vi "TrajectoryExecuteRelative.vi"(8 "Init":bool, 10 "End Relative\nOrientation Deg":dbl, 11 "Trajectory":T1 {"States"."POSE"."ROTATION"."SIN" format="%13.4f"; "States"."POSE"."ROTATION"."COS" format="%13.4f"; "States"."POSE"."ROTATION"."VALUE" format="%13.4f"; "States"."POSE"."TRANSLATION"."Y" format="%14.3f"; "States"."POSE"."TRANSLATION"."X" format="%14.3f"; "TotalTImeSecs" format="%20.3f"}) -> (0 "AtReference":bool, 2 "Done":bool, 3 "Chassis Velocity Target Met,Met,Rad":T6 {"vOmega" format="%10.3f"; "vY" format="%10.3f"; "vX" format="%10.3f"})   [LabVIEW 2023]
uses:
  <vilib>/Rock Robotics/WPI/ThirdParty/JAS_Junk/TrajLib/TypeDef/CHASSIS_SPEEDS.ctl
  <vilib>/Rock Robotics/WPI/ThirdParty/JAS_Junk/TrajLib/TypeDef/TRAJECTORY.ctl
  <vilib>/Rock Robotics/WPI/ThirdParty/JAS_Junk/TrajLib/TypeDef/TRAJ_STATE.ctl
  <vilib>/Rock Robotics/WPI/ThirdParty/JAS_Junk/TrajLib/TypeDef/POSE2D.ctl
  <vilib>/Rock Robotics/WPI/ThirdParty/JAS_Junk/TrajLib/TypeDef/TRANSLATION2D.ctl
  <vilib>/Rock Robotics/WPI/ThirdParty/JAS_Junk/TrajLib/TypeDef/ROTATION2D.ctl
  <vilib>/Rock Robotics/WPI/ThirdParty/JAS_Junk/TrajLib/VI/Util_GetTime_U32.vi
  <vilib>/Rock Robotics/WPI/ThirdParty/JAS_Junk/TrajLib/SwerveOdometry_UpdateX.vi
  <vilib>/Rock Robotics/WPI/ThirdParty/JAS_Junk/TrajLib/SwerveOdometry_ResetPosition.vi
  <vilib>/Rock Robotics/WPI/ThirdParty/JAS_Junk/TrajLib/SwerveOdometry_New.vi
  <vilib>/Rock Robotics/WPI/ThirdParty/JAS_Junk/TrajLib/HolDrvCtrl_New.vi
  <vilib>/Rock Robotics/WPI/ThirdParty/JAS_Junk/TrajLib/HolDrvCtrl_PackPID.vi
  <vilib>/Rock Robotics/WPI/ThirdParty/JAS_Junk/TrajLib/HolDrvCtrl_SetTolerance.vi
  <vilib>/Rock Robotics/WPI/ThirdParty/JAS_Junk/TrajLib/HolDrvCtrl_SetEnabled.vi
  <vilib>/Rock Robotics/WPI/ThirdParty/JAS_Junk/TrajLib/HolDrvCtrl_Calculate_Trajectory.vi
  <vilib>/Rock Robotics/WPI/ThirdParty/JAS_Junk/TrajLib/HolDrvCtrl_AtReference.vi
  <vilib>/Rock Robotics/WPI/ThirdParty/JAS_Junk/TrajLib/ProfiledPIDController_NewPeriod.vi
  <vilib>/Rock Robotics/WPI/ThirdParty/JAS_Junk/TrajLib/ProfiledPIDController_SetIntegratorRange.vi
  <vilib>/Rock Robotics/WPI/ThirdParty/JAS_Junk/TrajLib/ProfiledPIDController_DisableContInput.vi
  <vilib>/Rock Robotics/WPI/ThirdParty/JAS_Junk/TrajLib/ProfiledPIDController_EnableContInput.vi
  <vilib>/Rock Robotics/WPI/ThirdParty/JAS_Junk/TrajLib/TrapProfConstraint_New.vi
  <vilib>/Rock Robotics/WPI/ThirdParty/JAS_Junk/TrajLib/Translation2d_Create.vi
  <vilib>/Rock Robotics/WPI/ThirdParty/JAS_Junk/TrajLib/Rotation2d_Plus.vi
  <vilib>/Rock Robotics/WPI/ThirdParty/JAS_Junk/TrajLib/Twist2d_Create.vi
  <vilib>/Rock Robotics/WPI/ThirdParty/JAS_Junk/TrajLib/Rotation2d_Minus.vi
  <vilib>/Rock Robotics/WPI/ThirdParty/JAS_Junk/TrajLib/Pose2d_getTranslation.vi
  <vilib>/Rock Robotics/WPI/ThirdParty/JAS_Junk/TrajLib/Pose2d_New_TRRO.vi
  <vilib>/Rock Robotics/WPI/ThirdParty/JAS_Junk/TrajLib/VI/SwerveModulePosition_Get.vi
  <vilib>/Rock Robotics/WPI/ThirdParty/JAS_Junk/TrajLib/VI/SwerveModulePosition_New.vi
  <vilib>/Rock Robotics/WPI/ThirdParty/JAS_Junk/TrajLib/Twist2d_GetAll.vi
  <vilib>/Rock Robotics/WPI/ThirdParty/JAS_Junk/TrajLib/Pose2d_getRotation.vi
  <vilib>/Rock Robotics/SystemInterfaces/NetworkCommunication/NetComm_UsageReport_report.vi
  <vilib>/Rock Robotics/WPI/ThirdParty/JAS_Junk/TrajLib/PIDController_NewPeriod.vi
  <vilib>/Rock Robotics/WPI/ThirdParty/JAS_Junk/TrajLib/PIDController_SetIntegratorRange.vi
  <vilib>/Rock Robotics/WPI/ThirdParty/JAS_Junk/TrajLib/PIDController_Reset.vi
  <vilib>/Rock Robotics/WPI/ThirdParty/JAS_Junk/TrajLib/HolDrvCtrl_Calculate.vi
  <vilib>/Rock Robotics/WPI/ThirdParty/JAS_Junk/TrajLib/Pose2d_getXYAngle.vi
  <vilib>/Rock Robotics/WPI/ThirdParty/JAS_Junk/TrajLib/Rotation2d_GetRadians.vi
  <vilib>/Rock Robotics/WPI/ThirdParty/JAS_Junk/TrajLib/TrapProfState_New.vi
  <vilib>/Rock Robotics/WPI/ThirdParty/JAS_Junk/TrajLib/PIDController_DisableContinousInput.vi
  <vilib>/Rock Robotics/WPI/ThirdParty/JAS_Junk/TrajLib/PIDController_EnableContinousInput.vi
  <vilib>/Rock Robotics/WPI/ThirdParty/JAS_Junk/TrajLib/Rotation2d_RotateBy.vi
  <vilib>/Rock Robotics/WPI/ThirdParty/JAS_Junk/TrajLib/Rotation2d_UnaryMinus.vi
  <vilib>/Rock Robotics/WPI/ThirdParty/JAS_Junk/TrajLib/Rotation2d_GetAngleCosSin.vi
  <vilib>/Rock Robotics/WPI/ThirdParty/JAS_Junk/TrajLib/Pose2d_RelativeTo.vi
  <vilib>/Rock Robotics/WPI/ThirdParty/JAS_Junk/TrajLib/ProfiledPIDController_Calculate_Meas_Goal.vi
  <vilib>/Rock Robotics/WPI/ThirdParty/JAS_Junk/TrajLib/PIDController_Calculate_SP_PV.vi
  <vilib>/Rock Robotics/WPI/ThirdParty/JAS_Junk/TrajLib/ProfiledPIDController_Reset_PosOnly.vi
  <vilib>/Rock Robotics/WPI/ThirdParty/JAS_Junk/TrajLib/ChassisSpeeds_FromFieldRelativeSpeeds.vi
  <vilib>/Rock Robotics/WPI/ThirdParty/JAS_Junk/TrajLib/Rotation2d_CreateXY.vi
  <vilib>/Rock Robotics/WPI/ThirdParty/JAS_Junk/TrajLib/Transform2d_Create_PosePose.vi
  <vilib>/Rock Robotics/WPI/ThirdParty/JAS_Junk/TrajLib/ProfiledPIDController_SetGoal_PosOnly.vi
  <vilib>/Rock Robotics/WPI/ThirdParty/JAS_Junk/TrajLib/ProfiledPIDController_Calculate_Meas.vi
  <vilib>/Rock Robotics/WPI/ThirdParty/JAS_Junk/TrajLib/PIDController_SetSetpoint.vi
  <vilib>/Rock Robotics/WPI/ThirdParty/JAS_Junk/TrajLib/PIDController_Calculate_PV.vi
  <vilib>/Rock Robotics/WPI/ThirdParty/JAS_Junk/TrajLib/ProfiledPIDController_Reset.vi
  <vilib>/Rock Robotics/WPI/ThirdParty/JAS_Junk/TrajLib/Rotation2d_GetCos.vi
  <vilib>/Rock Robotics/WPI/ThirdParty/JAS_Junk/TrajLib/Rotation2d_GetSin.vi
  <vilib>/Rock Robotics/WPI/ThirdParty/JAS_Junk/TrajLib/Util_CalcDist.vi
  <vilib>/Rock Robotics/WPI/ThirdParty/JAS_Junk/TrajLib/Translation2d_RotateBy.vi
  <vilib>/Rock Robotics/WPI/ThirdParty/JAS_Junk/TrajLib/Translation2d_Minus.vi
  <vilib>/Rock Robotics/WPI/ThirdParty/JAS_Junk/TrajLib/ProfiledPIDController_SetGoal.vi
  <vilib>/Rock Robotics/WPI/ThirdParty/JAS_Junk/TrajLib/TrapProfile_New.vi
  <vilib>/Rock Robotics/WPI/ThirdParty/JAS_Junk/TrajLib/ProfiledPIDController_GetPeriod.vi
  <vilib>/Rock Robotics/WPI/ThirdParty/JAS_Junk/TrajLib/TrapProfile_Calculate.vi
  <vilib>/Rock Robotics/WPI/ThirdParty/JAS_Junk/TrajLib/ControllerUtil_GetModulusError.vi
  <vilib>/Rock Robotics/WPI/ThirdParty/JAS_Junk/TrajLib/TrapProfile_ShouldFlipAcceleration.vi
  <vilib>/Rock Robotics/WPI/ThirdParty/JAS_Junk/TrajLib/TrapProfile_Direct.vi
  <vilib>/Rock Robotics/WPI/ThirdParty/JAS_Junk/TrajLib/PIDController_GetPeriod.vi
  TrajectoryGlobals.vi
  <vilib>/Rock Robotics/SystemInterfaces/Utilities/FPGA_UtilitiesRead LocalTime.vi
  <vilib>/Rock Robotics/WPI/ThirdParty/JAS_Junk/TrajLib/VI/Util_GetTime_U64.vi
  <vilib>/Rock Robotics/WPI/ThirdParty/JAS_Junk/TrajLib/Globals/Util_LibraryGlobals.vi
  <vilib>/Rock Robotics/WPI/ThirdParty/JAS_Junk/TrajLib/VI/SwerveKinematics_ToTwist2dX.vi
  <vilib>/Rock Robotics/WPI/ThirdParty/JAS_Junk/TrajLib/Pose2d_Exp.vi
  <vilib>/Rock Robotics/WPI/ThirdParty/JAS_Junk/TrajLib/Trajectory_Library.lvlib
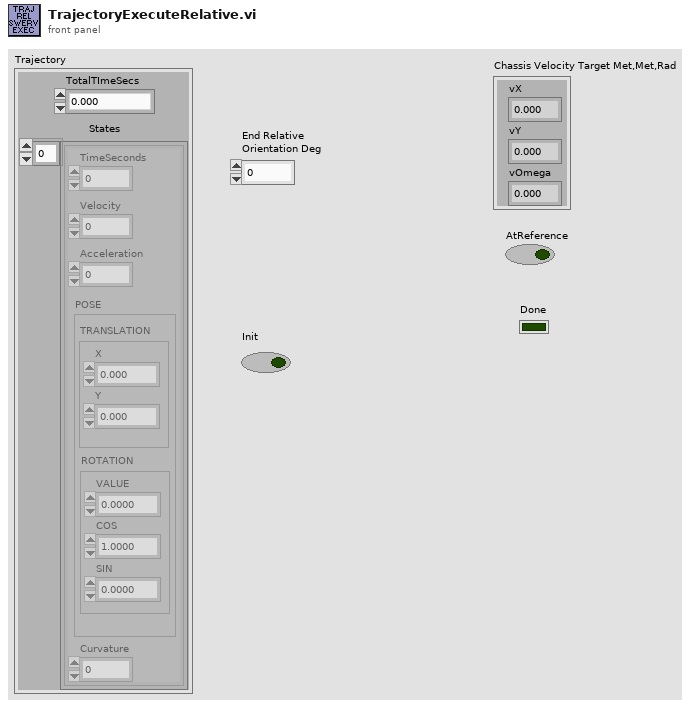
[diagram p1: front panel]
types:
  T1 = typedef "Trajectory_Library.lvlib/TRAJECTORY.ctl" = cluster{"TotalTImeSecs":dbl, "States":T2[]}
  T2 = typedef "Trajectory_Library.lvlib/TRAJ_STATE.ctl" = cluster{"TimeSeconds":dbl, "Velocity":dbl, "Acceleration":dbl, "POSE":T3, "Curvature":dbl}
  T3 = typedef "Trajectory_Library.lvlib/POSE2D.ctl" = cluster{"TRANSLATION":T4, "ROTATION":T5}
  T4 = typedef "Trajectory_Library.lvlib/TRANSLATION2D.ctl" = cluster{"X":dbl, "Y":dbl}
  T5 = typedef "Trajectory_Library.lvlib/ROTATION2D.ctl" = cluster{"VALUE":dbl, "COS":dbl, "SIN":dbl}
  T6 = typedef "Trajectory_Library.lvlib/CHASSIS_SPEEDS.ctl" = cluster{"vX":dbl, "vY":dbl, "vOmega":dbl}
  T7 = typedef "Trajectory_Library.lvlib/SWERVE_DRIVE_MODULE_POSITION.ctl" = cluster{"Distance":dbl, "Angle":T5, "P":bool}
  T8 = typedef "Trajectory_Library.lvlib/SWERVE_DRIVE_KINEMATICS.ctl" = cluster{"NumModules":i32, "InverseKinematics":T9, "ForwardKinematics":T9, "Modules":T4[], "PrevCoR":T4, "SavedModuleStates":T10[]}
  T9 = typedef "NI_Matrix.lvlib/RealMatrix.ctl" = dbl[][]
  T10 = typedef "Trajectory_Library.lvlib/SWERVE_DRIVE_MODULE_STATE.ctl" = cluster{"Speed":dbl, "Angle":T5}
  T11 = typedef "Trajectory_Library.lvlib/HOLONOMIC_PACK_TUNING.ctl" = cluster{"X PID Tuning":T12, "Y PID Tuning":T12, "thetaProfiledPID_CTRL":T13}
  T12 = typedef "Trajectory_Library.lvlib/PID_TUNING.ctl" = cluster{"Kp":dbl, "Ki":dbl, "Kd":dbl, "MaximumIntegral":dbl, "MinimumIntegral":dbl, "IntegralZone":dbl}
  T13 = typedef "Trajectory_Library.lvlib/PROFILED_PID_CONTROLLER.ctl" = cluster{"Controller":T14, "Goal":T15, "Setpoint":T15, "Constraint":T16}
  T14 = typedef "Trajectory_Library.lvlib/PID_CONTROLLER.ctl" = cluster{"Kp":dbl, "Ki":dbl, "Kd":dbl, "Period":dbl, "Max_Integral":dbl, "Min_Integral":dbl, "Max_Input":dbl, "Min_Input":dbl, "Continuous":bool, "PositionError":dbl, "VelocityError":dbl, "PrevError":dbl, "Total_Integral":dbl, "PositionTolerance":dbl, "VelocityTolerance":dbl, "SetPoint":dbl, "Kf":dbl, "Prev_Deriv":dbl, "Prev_Deriv 2":dbl, "DerivativeFilter":bool, "Min_Output":dbl, "Max_Output":dbl, "Prev_F_P":dbl, "Prev_F_P_2":dbl, "AntiWindupActive":bool, "Measurement":dbl, "IntegralZone":dbl}
  T15 = typedef "Trajectory_Library.lvlib/TRAPEZOID_PROFILE_STATE.ctl" = cluster{"Position":dbl, "Velocity":dbl}
  T16 = typedef "Trajectory_Library.lvlib/TRAPEZOID_PROFILE_CONSTRAINT.ctl" = cluster{"MaxVelocity":dbl, "MaxAcceleration":dbl}
  T17 = typedef "Trajectory_Library.lvlib/HOLONOMIC_DRV_CTRL.ctl" = cluster{"poseTolerance":T3, "poseError":T3, "Enabled":bool, "PID_xCtrl":T14, "PID_yCtrl":T14, "PROF_PID_thetaCtrl":T13, "RotationError":T5, "FirstRun":bool}
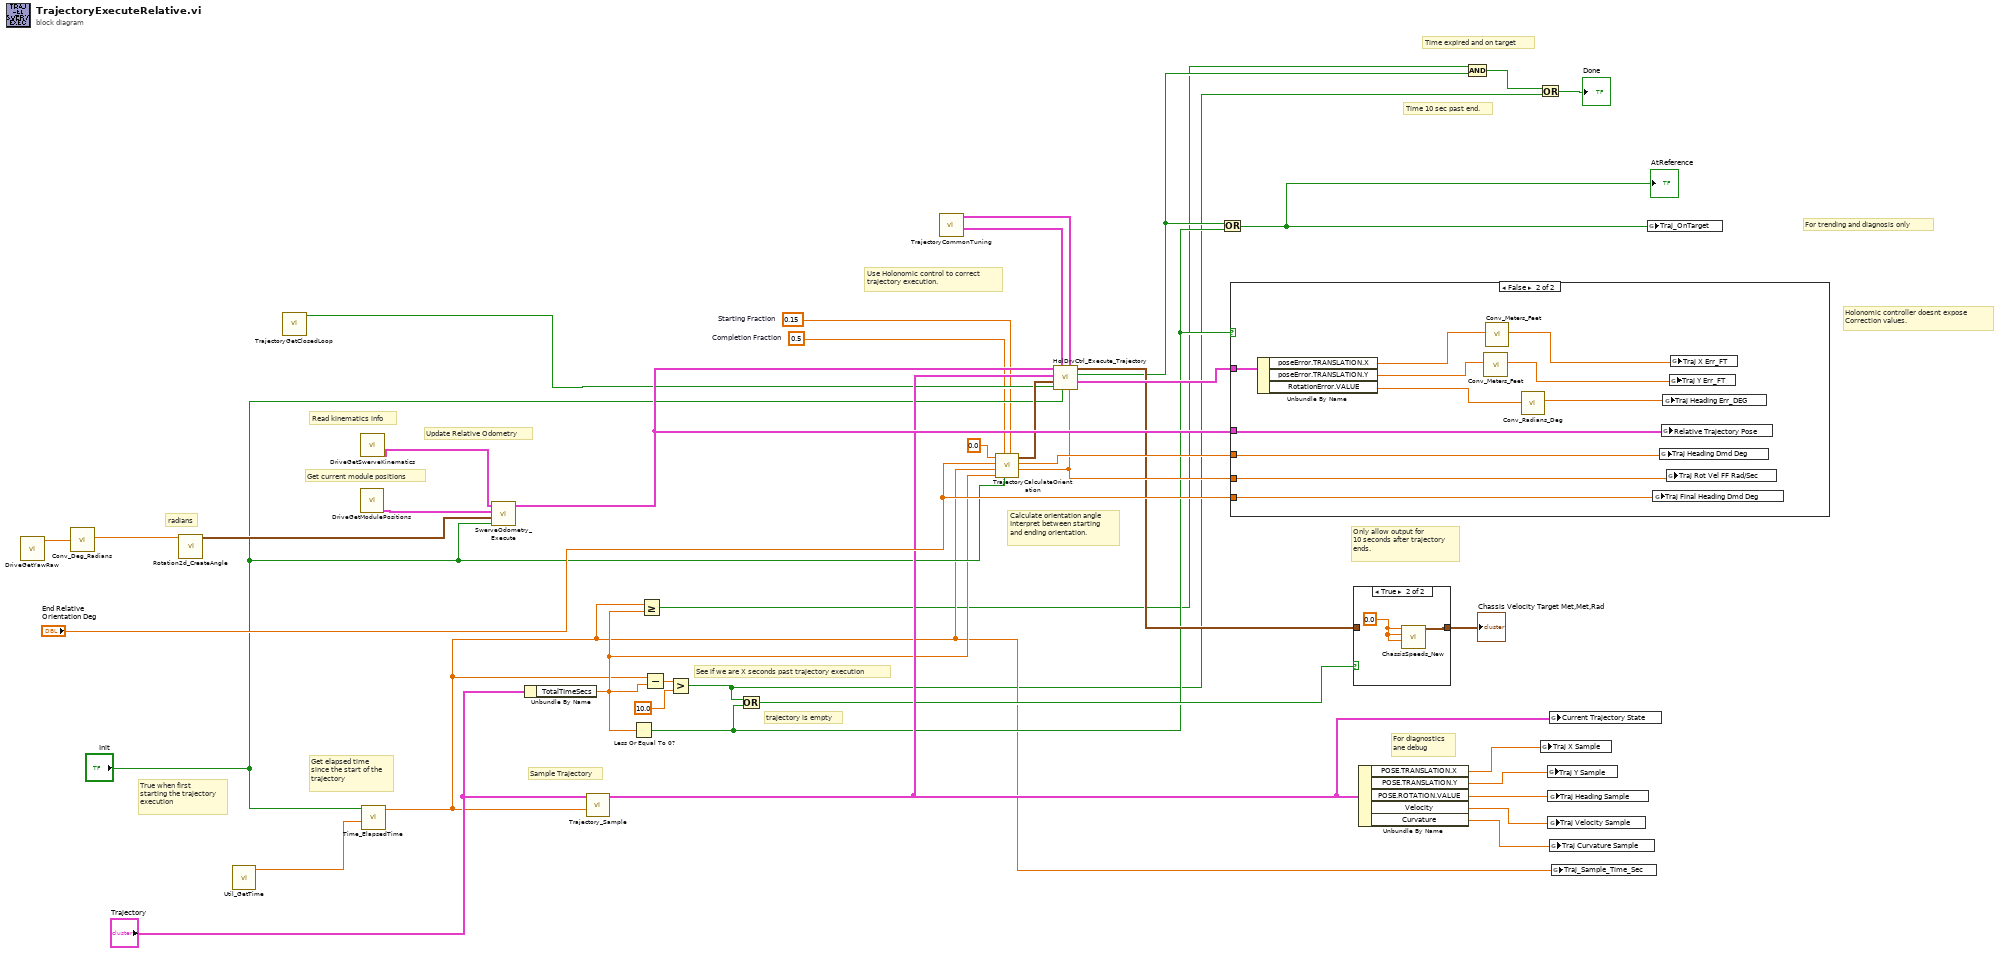
[diagram p0: block diagram]
diagram:
  w3 = 0.15  # Starting Fraction
  w4 = 0.5  # Completion Fraction
  # "Time 10 sec past end."
  # "Time expired and on target"
  # "trajectory is empty"
  # "Calculate orientation angle\nInterpret between starting\nand ending orientation."
  # "Get current module positions"
  # "True when first\nstarting the trajectory\nexecution"
  # "Get elapsed time\nsince the start of the\ntrajectory"
  # "Holonomic controller doesnt expose\nCorrection values."
  # "Use Holonomic control to correct\ntrajectory execution."
  # "For trending and diagnosis only"
  # "For diagnostics\nane debug"
  # "Update Relative Odometry"
  # "Read kinematics info"
  # "Sample Trajectory"
  # "See if we are X seconds past trajectory execution"
  # "radians"
  # "Only allow output for\n10 seconds after trajectory\nends."
  n1 = call "DriveGetYawRaw.vi"() -> ("YawRaw"=w14:dbl)  [unwired: 11 in]
  n2 = call <vilib>:"Conv_Deg_Radians.vi"("Degress"=w14) -> ("Radians"=w13:dbl)  [unwired: 10 in]
  n3 = call <vilib>:"Rotation2d_CreateAngle.vi"("Angle"=w13) -> ("ROTATION"=w37:T5)  [unwired: 10 in]
  n4 = call <vilib>:"Util_GetTime.vi"() -> ("FPGA_Time_Seconds"=w36:dbl)  [unwired: 9 in, 2 out]
  n5 = call "TrajectoryGetClosedLoop.vi"() -> ("AUTO_CLOSED_LOOP"=w17:bool)  [unwired: 11 in]
  n6 = call "DriveGetModulePositions.vi"() -> ("Swerve_Drive_Modual_Positions"=w15:T7[])  [unwired: 11 in]
  n7 = call "DriveGetSwerveKinematics.vi"() -> ("SWERVE_DRIVE_KINEMATICS"=w16:T8)  [unwired: 11 in]
  n8 = call <vilib>:"Time_ElapsedTime.vi"("PassthroughTime_SEC"=w36, "Reset"="Init") -> ("Elapsed Time Sec"=w10:dbl)  [unwired: 9 in]
  n9 = call <vilib>:"SwerveOdometry_Execute.vi"("Init"="Init", "Rotation"=w37, "Swerve Module Positions"=w15, "SWERVE_DRIVE_KINEMATICS"=w16) -> ("Current Pose"=w28:T3)  [unwired: 5 in, 2 out]
  n10 = Unbundle By Name("Trajectory") -> ("TotalTImeSecs"=w11:dbl)
  n11 = call <vilib>:"Trajectory_Sample.vi"("Time"=w10, "InputTRAJECTORY"="Trajectory") -> ("OutputTRAJ_STATE"=w23:T2)  [unwired: 9 in]
  n12 = Less Or Equal To 0?(x=w11) -> (x <= 0?=w19:bool)
  n13 = Greater Or Equal?(x=w10, y=w11) -> (x >= y?=w6:bool)
  n14 = Subtract(x=w10, y=w11) -> (x-y=w40:dbl)
  n15 = Greater?(x=w40, y=10.0) -> (0:w5:bool)
  n16 = Or(x=w5, y=w19) -> (x .or. y?=w21:bool)
  n17 = call "TrajectoryCommonTuning.vi"() -> ("out POSe"=w1:T3, "HOLONOMIC_CTRL_PACK_TUNING"=w2:T11)  [unwired: 10 in]
  n18 = call "TrajectoryCalculateOrientation.vi"("Starting Fraction"=w3, "Init"="Init", "Completion Fraction"=w4, "Total Trajectory Time Sec"=w11, "Elapsed Traj Time Sec"=w10, "End Orientation Demand DEG"="End Relative\nOrientation Deg", "Starting Orientation  DEG"=0.0) -> ("Rotational Velocity Rad Per Sec"=w25:dbl, "Orientation Demand Deg"=w30:dbl, "Orientation Demand"=w27:T5)  [unwired: 2 in]
  n19 = call <vilib>:"HolDrvCtrl_Execute_Trajectory.vi"("Rotational Velocity Feedforward \nRad/Sec"=w25, "HOLONOMIC_CTRL_PACK_TUNING"=w2, "Reset"="Init", "Tolerance"=w1, "Enable"=w17, "angleRef"=w27, "desiredTrajState"=w23, "currentPose"=w28) -> ("outHOLONOMIC_DRV_CTRL"=w26:T17, "AtReference"=w7:bool, "calcChassisSpeed"=w22:T6)  [unwired: 1 in]
  n20 = Or(x=w7, y=w19) -> (x .or. y?=w20:bool)
  "AtReference" <- w20
  n21 = case shown="False" w19 {
    tunnel: w30 -> [_ w51]
    tunnel: "End Relative\nOrientation Deg" -> [_ w50]
    tunnel: w28 -> [_ w44]
    tunnel: w26 -> [_ w43]
    tunnel: w25 -> [_ w42]
    frame True {
    }
    frame False {
      n22 = Unbundle By Name(w43) -> ("poseError.TRANSLATION.X"=w48:dbl, "poseError.TRANSLATION.Y"=w47:dbl, "RotationError.VALUE"=w41:dbl)
      n23 = call <vilib>:"Conv_Meters_Feet.vi"("Meters"=w47) -> ("Feet"=w46:dbl)  [unwired: 10 in]
      n24 = call <vilib>:"Conv_Meters_Feet.vi"("Meters"=w48) -> ("Feet"=w45:dbl)  [unwired: 10 in]
      n25 = call <vilib>:"Conv_Radians_Deg.vi"("Radians"=w41) -> ("Degrees"=w49:dbl)  [unwired: 10 in]
      n26 = global write "TrajectoryGlobals.vi" "Traj Final Heading Dmd Deg"(w50) -> ()
      n27 = global write "TrajectoryGlobals.vi" "Traj Heading Dmd Deg"(w51) -> ()
      n28 = global write "TrajectoryGlobals.vi" "Relative Trajectory Pose"(w44) -> ()
      n29 = global write "TrajectoryGlobals.vi" "Traj Heading Err_DEG"(w49) -> ()
      n30 = global write "TrajectoryGlobals.vi" "Traj Rot Vel FF Rad/Sec"(w42) -> ()
      n31 = global write "TrajectoryGlobals.vi" "Traj Y Err_FT"(w46) -> ()
      n32 = global write "TrajectoryGlobals.vi" "Traj X Err_FT"(w45) -> ()
    }
  }
  n33 = case shown="True" w21 {
    tunnel: w22 -> [w52 _]
    tunnel: [w52 w53] -> w38
    frame False {
    }
    frame True {
      w54 = 0.0 ("vX")
      n34 = call <vilib>:"ChassisSpeeds_New.vi"("vAngular"=w54, "vY"=w54, "vX"=w54) -> ("CHASSIS"=w53:T6)  [unwired: 8 in]
    }
  }
  "Chassis Velocity Target Met,Met,Rad" <- w38
  n35 = Unbundle By Name(w23) -> ("POSE.TRANSLATION.X"=w35:dbl, "POSE.TRANSLATION.Y"=w34:dbl, "POSE.ROTATION.VALUE"=w33:dbl, "Velocity"=w32:dbl, "Curvature"=w31:dbl)
  n36 = And(x=w6, y=w7) -> (x .and. y?=w9:bool)
  n37 = Or(x=w9, y=w5) -> (x .or. y?=→"Done":bool)
  n38 = global write "TrajectoryGlobals.vi" "Traj X Sample"(w35) -> ()
  n39 = global write "TrajectoryGlobals.vi" "Traj Y Sample"(w34) -> ()
  n40 = global write "TrajectoryGlobals.vi" "Traj Heading Sample"(w33) -> ()
  n41 = global write "TrajectoryGlobals.vi" "Traj Velocity Sample"(w32) -> ()
  n42 = global write "TrajectoryGlobals.vi" "Current Trajectory State"(w23) -> ()
  n43 = global write "TrajectoryGlobals.vi" "Traj Curvature Sample"(w31) -> ()
  n44 = global write "TrajectoryGlobals.vi" "Traj_Sample_Time_Sec"(w10) -> ()
  n45 = global write "TrajectoryGlobals.vi" "Traj_OnTarget"(w20) -> ()
